vi "Controls.vi"() -> ()   [LabVIEW 2010]
panel:
  in  "参数类型":T1(ring)
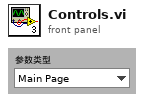
[diagram p1: front panel]
types:
  T1 = enum16{"Main Page", "Diagnostics", "Set Points", "Digital Inputs", "Control Outputs", "Digital Outputs", "Current Step", "Cascade"}
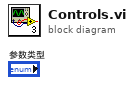
[diagram p0: block diagram]
diagram:
